vi "Start Simulation.vi"() -> (0 "Left Hem Path":path, 1 "Right Hem Path":path, 4 "TrainedPath":path, 6 "Action":enum16{"Trained", "Load", "New", "Cancel"}(ring))   [LabVIEW 2013]
panel:
  in  "Cancel Button":bool
  in  "NEW AER":bool
  in  "Trained AER":i32(listbox)
  in  "LOAD AER":bool
  # "Saved Configuration Files"
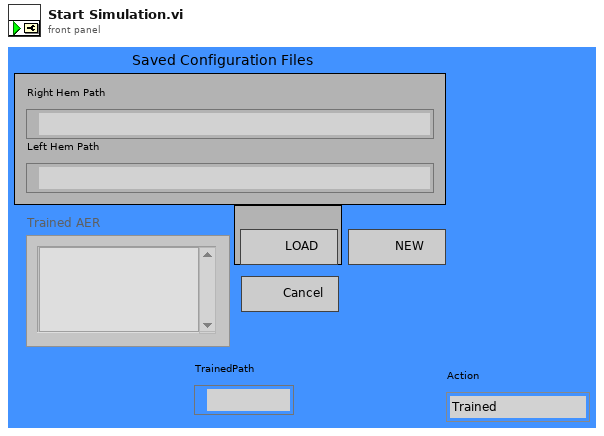
[diagram p1: front panel]
types:
  T1 = enum16{"open", "replace", "create", "open or create", "replace or create", "replace or create with confirmation"}
  T2 = enum8{"Enabled", "Disabled", "Disabled and Grayed Out"}
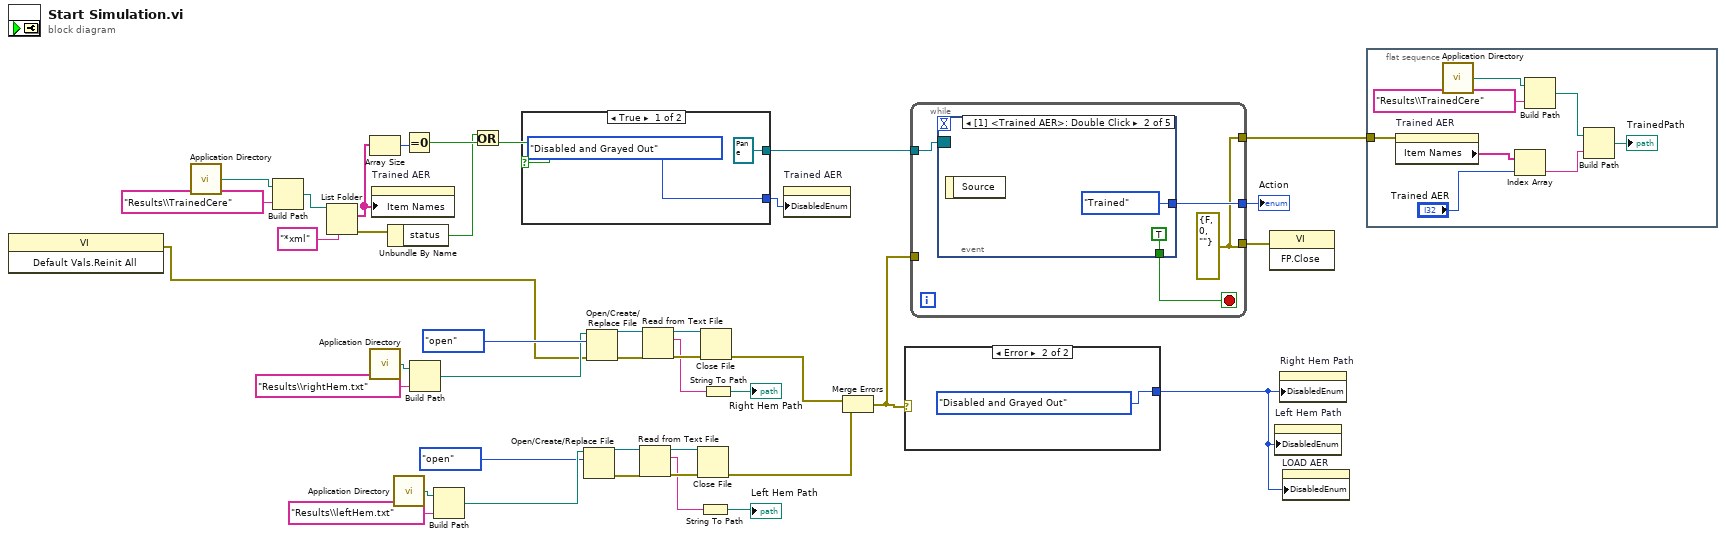
[diagram p0: block diagram]
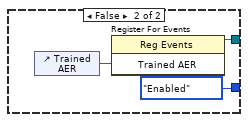
[diagram p2: hidden frame]
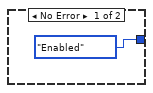
[diagram p3: hidden frame]
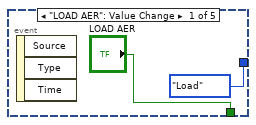
[diagram p4: hidden frame]
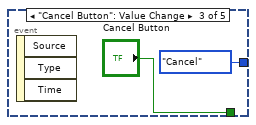
[diagram p5: hidden frame]
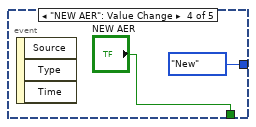
[diagram p6: hidden frame]
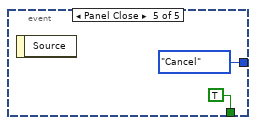
[diagram p7: hidden frame]
diagram:
  n1 = invoke class="VI" method="Default Vals.Reinit All"() -> (error out=w1:errorcluster)  [unwired: 3 in, 2 out]
  n2 = call <vilib>:"Application Directory.vi"() -> ("Application Directory"=w14:path)
  n3 = Build Path(base path=w14, name or relative path="Results\\TrainedCere") -> (appended path=w16:path)
  n4 = List Folder(path=w16, pattern="*xml") -> (filenames=w12:string[], error out=w4:errorcluster)  [unwired: 2 in, 2 out]
  n5 = Array Size(array=w12) -> (size(s)=w11:i32)
  n6 = call <vilib>:"Application Directory.vi"() -> ("Application Directory"=w39:path)
  n7 = property on="Trained AER" class="LstBox (strict)"("Item Names"=w12) -> ()  [unwired: 2 in, 2 out]
  n8 = Unbundle By Name(w4) -> ("status"=w2:bool)
  n9 = call <vilib>:"Application Directory.vi"() -> ("Application Directory"=w25:path)
  n10 = Equal To 0?(x=w11) -> (x = 0?=w10:bool)
  n11 = Build Path(base path=w39, name or relative path="Results\\rightHem.txt") -> (appended path=w37:path)
  n12 = Build Path(base path=w25, name or relative path="Results\\leftHem.txt") -> (appended path=w27:path)
  n13 = Or(x=w2, y=w10) -> (x .or. y?=w3:bool)
  n14 = case shown="True" w3 {
    tunnel: [refnum<event-registration> refnum ("Event Registration Refnum") w44] -> w9
    tunnel: [T2."Disabled and Grayed Out" ("Disabled") T2."Enabled" ("Disabled")] -> w5
    frame True {
    }
    frame False {
      n15 = control-ref of="Trained AER"() -> (w45:refnum<vi>)
      n16 = register-events(w45) -> (reference out=w44:refnum<event-registration>)  [unwired: 2 in, 1 out]
    }
  }
  n17 = Open/Create/Replace File(file path (use dialog)=w27, operation (0:open)=T1."open") -> (refnum out=w29:refnum<file>, error out=w28:errorcluster)  [unwired: 4 in, 1 out]
  n18 = Open/Create/Replace File(file path (use dialog)=w37, error in=w1, operation (0:open)=T1."open") -> (refnum out=w35:refnum<file>, error out=w36:errorcluster)  [unwired: 3 in, 1 out]
  n19 = Read from Text File(file (use dialog)=w29, error in=w28) -> (refnum out=w30:refnum<file>, text=w21:string, error out=w31:errorcluster)  [unwired: 2 in, 1 out]
  n20 = Read from Text File(file (use dialog)=w35, error in=w36) -> (refnum out=w34:refnum<file>, text=w22:string, error out=w33:errorcluster)  [unwired: 2 in, 1 out]
  n21 = Close File(refnum=w30, error in=w31) -> (error out=w19:errorcluster)  [unwired: 1 out]
  n22 = String To Path(string=w21) -> (path=→"Left Hem Path":path)
  n23 = Close File(refnum=w34, error in=w33) -> (error out=w20:errorcluster)  [unwired: 1 out]
  n24 = String To Path(string=w22) -> (path=→"Right Hem Path":path)
  n25 = property on="Trained AER" class="LstBox (strict)"("DisabledEnum"=w5) -> ()  [unwired: 2 in, 2 out]
  n26 = Merge Errors(w20, w19) -> (w13:errorcluster)
  n27 = case shown="Error" w13 {
    tunnel: [T2."Enabled" ("Disabled") T2."Disabled and Grayed Out" ("Disabled")] -> w6
    frame No Error {
    }
    frame Error {
    }
  }
  n28 = while {
    tunnel: [w50] -> w18
    tunnel: w13 -> [_]
    tunnel: w9 -> [w49]
    tunnel: [w48] -> w8
    tunnel: [w48] -> w7
    stop <- w51 stop-if-true
    w48 = errorcluster {"status"=FALSE, "code"=0, "source"=""} ("error out")
    n29 = event shown="[1] <Trained AER>: Double Click" {
      selector: w49 -> [_ _ _ _ _]
      dyn-events: _ -> [_ _ _ _ _]
      timeout: _ -> [_ _ _ _ _]
      tunnel: ["LOAD AER" TRUE ("NEW AER") "Cancel Button" "NEW AER" TRUE] -> w51
      tunnel: [enum16{"Trained", "Load", "New", "Cancel"}."Load" enum16{"Trained", "Load", "New", "Cancel"}."Trained" enum16{"Trained", "Load", "New", "Cancel"}."Cancel" enum16{"Trained", "Load", "New", "Cancel"}."New" enum16{"Trained", "Load", "New", "Cancel"}."Cancel"] -> w50
      event "LOAD AER": Value Change {
        n30 = event-data() -> ()  [unwired: 1 in, 3 out]
      }
      event Double Click {
        n31 = event-data() -> ()  [unwired: 1 in, 1 out]
      }
      event "Cancel Button": Value Change {
        n32 = event-data() -> ()  [unwired: 1 in, 3 out]
      }
      event "NEW AER": Value Change {
        n33 = event-data() -> ()  [unwired: 1 in, 3 out]
      }
      event Panel Close {
        n34 = event-data() -> ()  [unwired: 1 in, 1 out]
      }
    }
  }
  "Action" <- w18
  n35 = invoke class="VI" method="FP.Close"(error in=w8) -> ()  [unwired: 2 in, 3 out]
  n36 = property on="Left Hem Path" class="Path"("DisabledEnum"=w6) -> ()  [unwired: 2 in, 2 out]
  n37 = property on="Right Hem Path" class="Path"("DisabledEnum"=w6) -> ()  [unwired: 2 in, 2 out]
  n38 = property on="LOAD AER" class="Bool"("DisabledEnum"=w6) -> ()  [unwired: 2 in, 2 out]
  n39 = flat-sequence {
    tunnel: w7 -> [w62]
    frame #0 {
      n40 = property on="Trained AER" class="LstBox (strict)"(error in=w62) -> ("Item Names"=w69:string[])  [unwired: 1 in, 2 out]
      n41 = call <vilib>:"Application Directory.vi"() -> ("Application Directory"=w66:path)
      n42 = Index Array(array=w69, index="Trained AER") -> (element=w64:string)
      n43 = Build Path(base path=w66, name or relative path="Results\\TrainedCere") -> (appended path=w65:path)
      n44 = Build Path(base path=w65, name or relative path=w64) -> (appended path=→"TrainedPath":path)
    }
  }
